vi "Value Pair Grid Visible Read.vi"(8 "error in (no error)":errorcluster, 11 "3D Plot.lvclass in":refnum<class "3D Plot.lvclass">) -> (0 "error out":errorcluster, 1 "Show Grid?":bool, 3 "3D Plot.lvclass out":refnum<class "3D Plot.lvclass">)   [LabVIEW 2020, in "3D Plot.lvclass"]
uses:
  3D Plot.lvclass
  3D Plot.lvclass/3D Plot.ctl
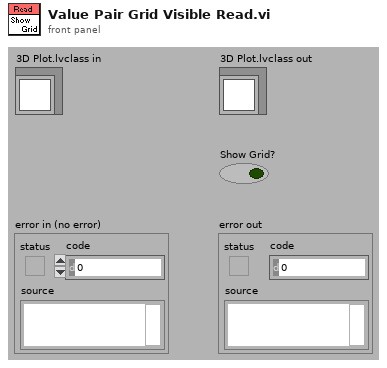
[diagram p1: front panel]
types:
  T1 = typedef "3D Plot.lvclass/Value Pair Property.ctl" = T2[]
  T2 = typedef "3D Plot.lvclass/Value Pair Cluster.ctl" = cluster{"Value Pair Array":cluster{"Value":sgl, "Name":string}[], "Show Tick":bool, "Show Grid":bool, " Label Mode":enum16{"Name", "Value", "None"}}
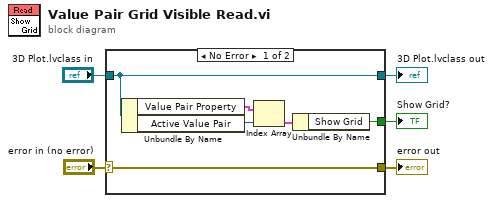
[diagram p0: block diagram]
diagram:
  n1 = case shown="No Error" "error in (no error)" {
    selector: "error in (no error)" -> [w10 w12]
    tunnel: [w6 _] -> w5
    tunnel: "3D Plot.lvclass in" -> [w11 w13]
    tunnel: [w11 w13] -> w3
    tunnel: [w10 w12] -> w1
    frame No Error {
      n2 = Unbundle By Name(w11) -> ("Value Pair Property"=w9:T1, "Active Value Pair"=w8:enum16{"X-axis", "Y-axis", "Z-axis"})
      n3 = Index Array(array=w9, index=w8) -> (element=w7:T2)
      n4 = Unbundle By Name(w7) -> ("Show Grid"=w6:bool)
    }
    frame Error {
    }
  }
  "error out" <- w1
  "Show Grid?" <- w5
  "3D Plot.lvclass out" <- w3
